vi "Route Triggers Impl.vi"(0 "trigger routes":T2(array[cluster]) {"pxi trigger number" items=["VXI/PXI TTL Line 0"=0, "VXI/PXI TTL Line 1"=1, "VXI/PXI TTL Line 2"=2, "VXI/PXI TTL Line 3"=3, "VXI/PXI TTL Line 4"=4, "VXI/PXI TTL Line 5"=5, "VXI/PXI TTL Line 6"=6, "VXI/PXI TTL Line 7"=7, "VXI ECL Line 0"=8, "VXI ECL Line 1"=9, "Front Panel Input"=27, "Front Panel Output"=28]}, 2 "map(T)/unmap(F)":bool=TRUE, 11 "error in":errorcluster) -> (15 "error out":errorcluster)   [LabVIEW 2019]
uses:
  <vilib>/Instr/_visa.llb/VISA Unmap Trigger Trigger Source.ctl
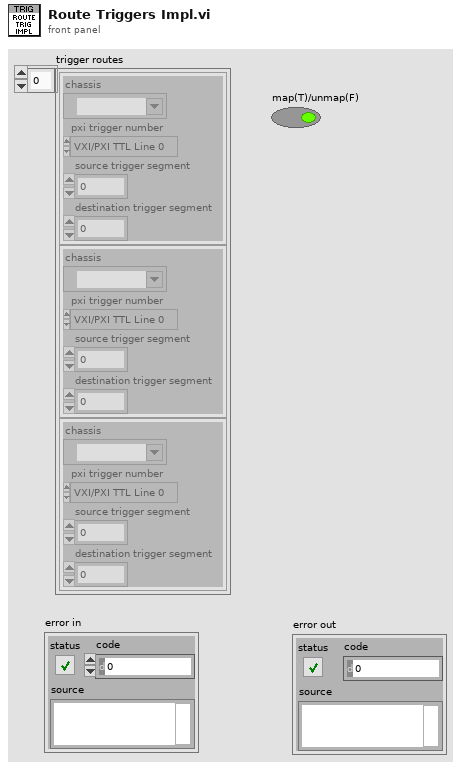
[diagram p1: front panel]
types:
  T1 = typedef "VISA Unmap Trigger Trigger Source.ctl" = i16
  T2 = cluster{"chassis":refnum<visa-resource-name>, "pxi trigger number":T1, "source trigger segment":i16, "destination trigger segment":i16}[]
  T3 = cluster{"trigger route":cluster{"chassis":refnum<visa-resource-name>, "pxi trigger number":T1, "source trigger segment":i16, "destination trigger segment":i16}, "map?":bool}[]
  T4 = cluster{"trigger route":cluster{"chassis":refnum<visa-resource-name>, "pxi trigger number":T1, "source trigger segment":i16, "destination trigger segment":i16}, "map?":bool}
  T5 = cluster{"chassis":refnum<visa-resource-name>, "pxi trigger number":T1, "source trigger segment":i16, "destination trigger segment":i16}
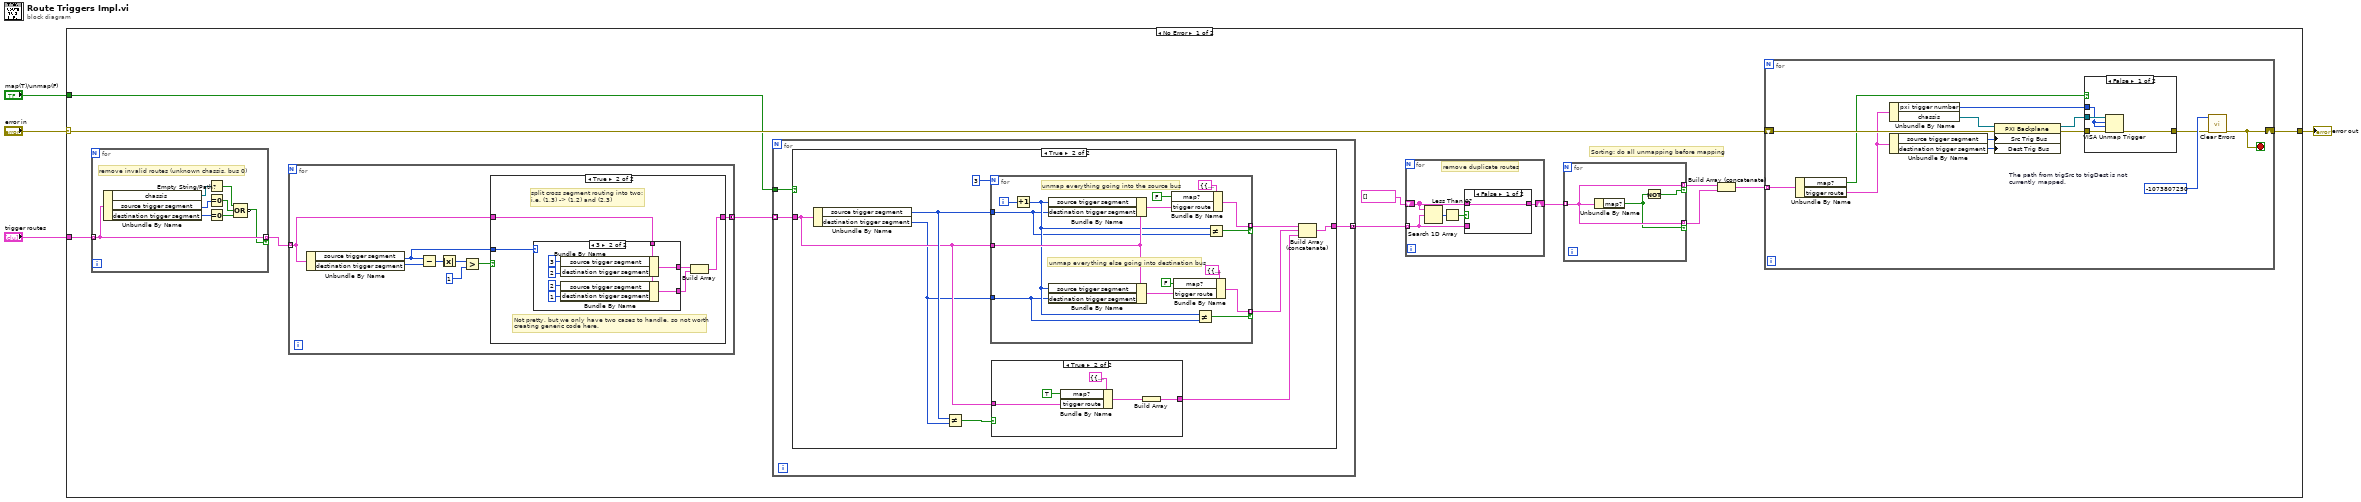
[diagram p0: block diagram]
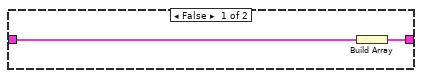
[diagram p2: hidden frame]
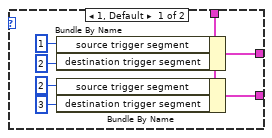
[diagram p3: hidden frame]
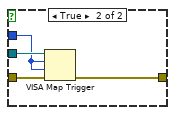
[diagram p4: hidden frame]
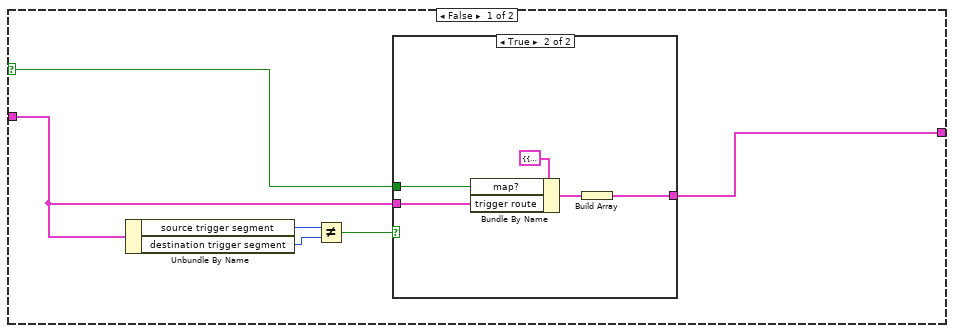
[diagram p5: hidden frame]
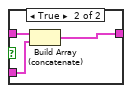
[diagram p8: hidden frame]
diagram:
  n1 = case shown="No Error" "error in" {
    selector: "error in" -> [w16 w130]
    tunnel: [w15 w130] -> w4
    tunnel: "map(T)/unmap(F)" -> [w14 _]
    tunnel: "trigger routes" -> [w12 _]
    frame No Error {
      # "Sorting: do all unmapping before mapping"
      n2 = for {
        tunnel: w12 -> [w53] mode=indexing
        tunnel: [w53] -> w6 mode=indexing if=w46
        # "remove invalid routes (unknown chassis, bus 0)"
        n3 = Unbundle By Name(w53) -> ("chassis"=w49:refnum<visa-resource-name>, "source trigger segment"=w51:i16, "destination trigger segment"=w52:i16)
        n4 = Empty String/Path?(string/path=w49) -> (empty?=w48:bool)
        n5 = Equal To 0?(x=w51) -> (x = 0?=w50:bool)
        n6 = Equal To 0?(x=w52) -> (x = 0?=w47:bool)
        n7 = Compound Arithmetic op=OR(w48, w50, w47) -> (invert w46:bool)
      }
      n8 = for {
        tunnel: w6 -> [w19] mode=indexing
        tunnel: [w18] -> w13 mode=concatenating
        n9 = Unbundle By Name(w19) -> ("source trigger segment"=w17:i16, "destination trigger segment"=w24:i16)
        n10 = Subtract(x=w17, y=w24) -> (x-y=w22:i16)
        n11 = Absolute Value(x=w22) -> (abs(x)=w21:i16)
        n12 = Greater?(x=w21, y=i16 1) -> (0:w20:bool)
        n13 = case shown="True" w20 {
          tunnel: w19 -> [w26 w31]
          tunnel: [w25 w27] -> w18
          tunnel: w17 -> [_ w30]
          frame False {
            n14 = Build Array(w26) -> (w25:T2)
          }
          frame True {
            # "Not pretty, but we only have two cases to handle, so not worth\ncreating generic code here."
            # "split cross segment routing into two:\ni.e. (1,3) -> (1,2) and (2,3)"
            n15 = case shown="3" w30 {
              tunnel: w31 -> [w33 w40]
              tunnel: [w34 w41] -> w29
              tunnel: [w32 w39] -> w28
              frame 1, Default {
                n16 = Bundle By Name(cluster=w33, "source trigger segment"=i16 1, "destination trigger segment"=i16 2) -> (w34:T5)
                n17 = Bundle By Name(cluster=w33, "source trigger segment"=i16 2, "destination trigger segment"=i16 3) -> (w32:T5)
              }
              frame 3 {
                n18 = Bundle By Name(cluster=w40, "source trigger segment"=i16 3, "destination trigger segment"=i16 2) -> (w41:T5)
                n19 = Bundle By Name(cluster=w40, "source trigger segment"=i16 2, "destination trigger segment"=i16 1) -> (w39:T5)
              }
            }
            n20 = Build Array(w29, w28) -> (w27:T2)
          }
        }
      }
      n21 = for {
        tunnel: w14 -> [w76]
        tunnel: w13 -> [w77] mode=indexing
        tunnel: [w75] -> w10 mode=concatenating
        n22 = case shown="True" w76 {
          selector: w76 -> [w83 _]
          tunnel: w77 -> [w79 w96]
          tunnel: [w82 w95] -> w75
          frame False {
            n23 = Unbundle By Name(w79) -> ("source trigger segment"=w81:i16, "destination trigger segment"=w80:i16)
            n24 = Not Equal?(x=w81, y=w80) -> (x != y?=w78:bool)
            n25 = case shown="True" w78 {
              tunnel: w83 -> [_ w87]
              tunnel: [_ w85] -> w82
              tunnel: w79 -> [_ w84]
              frame False {
                # "There is nothing to unmap within one bus...\n\nUnmap should be used for clean up operation (or after a succesfull map), we won't be unmapping any route within going in/out this bus.\n\nTo use a trigger within a bus, set the 'map' boolean to TRUE instead."
              }
              frame True {
                n26 = Bundle By Name(cluster=T4 {"trigger route"={"chassis"="", "pxi trigger number"=0, "source trigger segment"=0, "destination trigger segment"=0}, "map?"=TRUE}, "map?"=w87, "trigger route"=w84) -> (w86:T4)
                n27 = Build Array(w86) -> (w85:T3)
              }
            }
          }
          frame True {
            n28 = Unbundle By Name(w96) -> ("source trigger segment"=w97:i16, "destination trigger segment"=w90:i16)
            n29 = Not Equal?(x=w97, y=w90) -> (x != y?=w94:bool)
            n30 = for {
              N: 3 -> [_]
              tunnel: w96 -> [w104]
              tunnel: [w109] -> w93 mode=indexing if=w99
              tunnel: w97 -> [w101]
              tunnel: w90 -> [w98]
              tunnel: [w103] -> w92 mode=indexing if=w100
              i -> [w108]
              # "unmap everything else going into destination bus"
              # "unmap everything going into the source bus"
              n31 = Increment(x=w108) -> (x+1=w102:i32)
              n32 = Bundle By Name(cluster=w104, "source trigger segment"=w102, "destination trigger segment"=w101) -> (w111:T5)
              n33 = Bundle By Name(cluster=w104, "source trigger segment"=w102, "destination trigger segment"=w98) -> (w106:T5)
              n34 = Bundle By Name(cluster=T4 {"trigger route"={"chassis"="", "pxi trigger number"=0, "source trigger segment"=0, "destination trigger segment"=0}, "map?"=TRUE}, "map?"=FALSE, "trigger route"=w111) -> (w109:T4)
              n35 = Bundle By Name(cluster=T4 {"trigger route"={"chassis"="", "pxi trigger number"=0, "source trigger segment"=0, "destination trigger segment"=0}, "map?"=TRUE}, "map?"=FALSE, "trigger route"=w106) -> (w103:T4)
              n36 = Not Equal?(x=w102, y=w98) -> (x != y?=w100:bool)
              n37 = Not Equal?(x=w102, y=w101) -> (x != y?=w99:bool)
            }
            n38 = case shown="True" w94 {
              tunnel: w96 -> [_ w116]
              tunnel: [_ w113] -> w91
              frame False {
                # "same src and dest, no need to map within itself"
              }
              frame True {
                n39 = Bundle By Name(cluster=T4 {"trigger route"={"chassis"="", "pxi trigger number"=0, "source trigger segment"=0, "destination trigger segment"=0}, "map?"=TRUE}, "map?"=TRUE, "trigger route"=w116) -> (w114:T4)
                n40 = Build Array(w114) -> (w113:T3)
              }
            }
            n41 = Build Array (concatenate)(w93, w92, w91) -> (w95:T3)
          }
        }
      }
      n42 = for {
        shift-right: [w121] -> w9
        shift-left: T3 [] ("Array") -> [w122]
        tunnel: w10 -> [w123] mode=indexing
        # "remove duplicate routes"
        n43 = Search 1D Array(1D array=w122, element=w123) -> (index of element=w125:i32)  [unwired: 1 in]
        n44 = Less Than 0?(x=w125) -> (x < 0?=w124:bool)
        n45 = case shown="False" w124 {
          tunnel: w122 -> [w126 w129]
          tunnel: w123 -> [_ w128]
          tunnel: [w126 w127] -> w121
          frame False {
          }
          frame True {
            n46 = Build Array (concatenate)(w129, w128) -> (w127:T3)
          }
        }
      }
      n47 = for {
        tunnel: w9 -> [w120] mode=indexing
        tunnel: [w120] -> w8 mode=indexing if=w119
        tunnel: [w120] -> w5 mode=indexing if=w118
        n48 = Unbundle By Name(w120) -> ("map?"=w118:bool)
        n49 = Not(x=w118) -> (.not. x?=w119:bool)
      }
      n50 = Build Array (concatenate)(w8, w5) -> (w7:T3)
      n51 = for {
        shift-right: [w64] -> w15
        shift-left: w16 -> [w66]
        tunnel: w7 -> [w65] mode=indexing
        stop <- w64 stop-if-true
        w55 = -1073807250  # The path from trigSrc to trigDest is not currently mapped.
        n52 = Unbundle By Name(w65) -> ("map?"=w57:bool, "trigger route"=w56:T5)
        n53 = Unbundle By Name(w56) -> ("pxi trigger number"=w59:T1, "chassis"=w58:refnum<visa-resource-name>)
        n54 = Unbundle By Name(w56) -> ("source trigger segment"=w63:i16, "destination trigger segment"=w62:i16)
        n55 = property class="PXI Backplane"(reference=w58, error in=w66, "Src Trig Bus"=w63, "Dest Trig Bus"=w62) -> (reference out=w60:refnum<visa-resource-name>, error out=w61:errorcluster)
        n56 = case shown="False" w57 {
          tunnel: w61 -> [w70 w74]
          tunnel: w60 -> [w69 w73]
          tunnel: w59 -> [w68 w72]
          tunnel: [w67 w71] -> w54
          frame False {
            n57 = VISA Unmap Trigger(8:w70, 9:w68, 10:w68, 11:w69) -> (0:w67:errorcluster)  [unwired: 1 out]
          }
          frame True {
            n58 = VISA Map Trigger(8:w74, 9:w72, 10:w72, 11:w73) -> (0:w71:errorcluster)  [unwired: 1 in, 1 out]
          }
        }
        n59 = call <vilib>:"Clear Errors.vi"("error in (no error)"=w54, "specific error code to clear (0: all)"=w55) -> ("error out"=w64:errorcluster)  [unwired: 4 in, 1 out]
      }
    }
    frame Error {
    }
  }
  "error out" <- w4
